vi "LarmorOptimization(SubVI).vi"(10 "Initial Larmor Frequency":dbl, 11 "Pulse Train File in":path) -> (3 "Larmor Frequency 3":dbl)   [LabVIEW 2020]
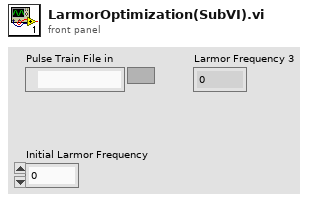
[diagram p1: front panel]
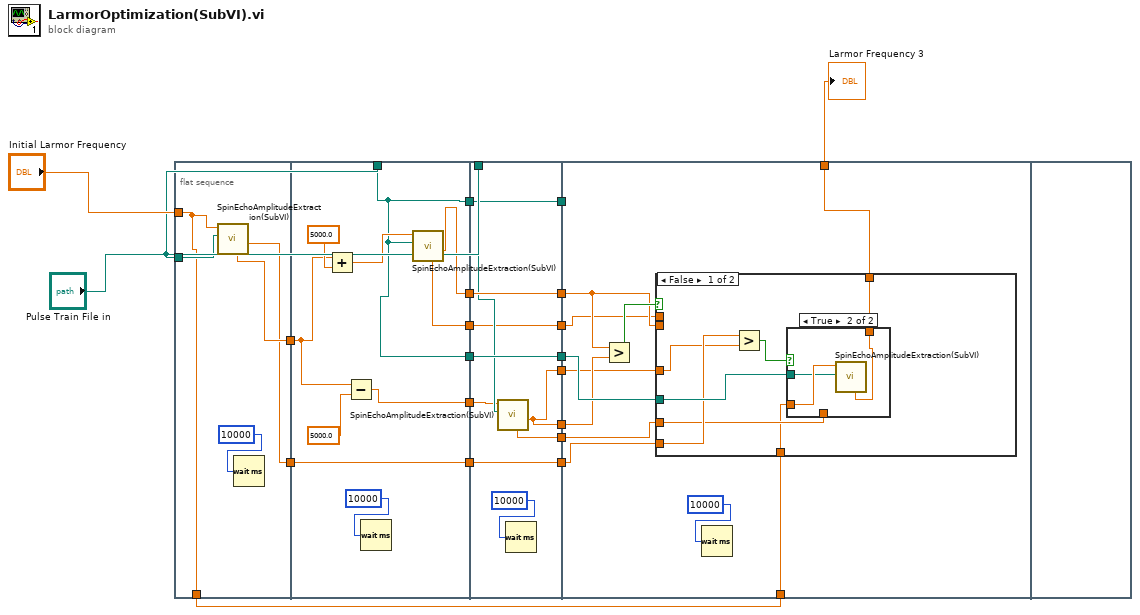
[diagram p0: block diagram]
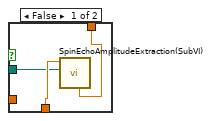
[diagram p2: hidden frame]
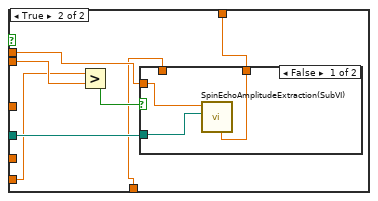
[diagram p3: hidden frame]
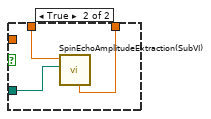
[diagram p4: hidden frame]
diagram:
  n1 = flat-sequence {
    tunnel: "Pulse Train File in" -> [w25]
    tunnel: "Initial Larmor Frequency" -> [w24]
    tunnel: [w23] -> w20
    tunnel: [w24] -> w1
    tunnel: [w21] -> w2
    tunnel: w20 -> [w34]
    tunnel: [w30] -> w19
    tunnel: "Pulse Train File in" -> [w31]
    tunnel: [w31] -> w18
    tunnel: [w31] -> w17
    tunnel: [w29] -> w16
    tunnel: [w27] -> w15
    tunnel: [w26] -> w3
    tunnel: w2 -> [w26]
    tunnel: w19 -> [w45]
    tunnel: [w45] -> w14
    tunnel: [w37] -> w13
    tunnel: w18 -> [w44]
    tunnel: [w44] -> w12
    tunnel: w17 -> [w43]
    tunnel: [w43] -> w11
    tunnel: "Pulse Train File in" -> [w42]
    tunnel: w16 -> [w41]
    tunnel: [w39] -> w10
    tunnel: w15 -> [w39]
    tunnel: [w38] -> w9
    tunnel: [w37] -> w5
    tunnel: [w36] -> w4
    tunnel: w3 -> [w36]
    tunnel: w14 -> [w47]
    tunnel: w13 -> [w54]
    tunnel: w12 -> [w55]
    tunnel: w11 -> [_]
    tunnel: w10 -> [w46]
    tunnel: w9 -> [w50]
    tunnel: [w53] -> w7
    tunnel: w5 -> [w51]
    tunnel: w4 -> [w49]
    tunnel: w1 -> [w48]
    frame #0 {
      n2 = call "SpinEchoAmplitudeExtraction(SubVI).vi"("Pulse Train File in"=w25, "Larmor Frequency in"=w24) -> ("Y value"=w21:dbl, "Larmor Frequency 3"=w23:dbl)  [unwired: 5 in, 3 out]
      n3 = Wait (ms)(milliseconds to wait=u32 10000) -> ()  [unwired: 1 out]
    }
    frame #1 {
      n4 = Add(x=w34, y=5000.0) -> (x+y=w32:dbl)
      n5 = Subtract(x=w34, y=5000.0) -> (x-y=w29:dbl)
      n6 = Wait (ms)(milliseconds to wait=u32 10000) -> ()  [unwired: 1 out]
      n7 = call "SpinEchoAmplitudeExtraction(SubVI).vi"("Pulse Train File in"=w31, "Larmor Frequency in"=w32) -> ("Y value"=w30:dbl, "Larmor Frequency 3"=w27:dbl)  [unwired: 5 in, 3 out]
    }
    frame #2 {
      n8 = call "SpinEchoAmplitudeExtraction(SubVI).vi"("Pulse Train File in"=w42, "Larmor Frequency in"=w41) -> ("Y value"=w37:dbl, "Larmor Frequency 3"=w38:dbl)  [unwired: 5 in, 3 out]
      n9 = Wait (ms)(milliseconds to wait=u32 10000) -> ()  [unwired: 1 out]
    }
    frame #3 {
      n10 = Greater?(x=w47, y=w54) -> (0:w56:bool)
      n11 = case shown="False" w56 {
        tunnel: w49 -> [w61 w73]
        tunnel: w55 -> [w62 w75]
        tunnel: w47 -> [_ w74]
        tunnel: w51 -> [w59 _]
        tunnel: [w60 w72] -> w53
        tunnel: w50 -> [w58 _]
        tunnel: w48 -> [w57 w70]
        tunnel: w46 -> [_ w71]
        frame False {
          n12 = Greater?(x=w61, y=w59) -> (0:w63:bool)
          n13 = case shown="True" w63 {
            tunnel: w62 -> [w65 w68]
            tunnel: w57 -> [_ w69]
            tunnel: [w64 w67] -> w60
            tunnel: w58 -> [w66 _]
            frame False {
              n14 = call "SpinEchoAmplitudeExtraction(SubVI).vi"("Pulse Train File in"=w65, "Larmor Frequency in"=w66) -> ("Larmor Frequency 3"=w64:dbl)  [unwired: 5 in, 4 out]
            }
            frame True {
              n15 = call "SpinEchoAmplitudeExtraction(SubVI).vi"("Pulse Train File in"=w68, "Larmor Frequency in"=w69) -> ("Larmor Frequency 3"=w67:dbl)  [unwired: 5 in, 4 out]
            }
          }
        }
        frame True {
          n16 = Greater?(x=w73, y=w74) -> (0:w76:bool)
          n17 = case shown="False" w76 {
            tunnel: w75 -> [w78 w80]
            tunnel: w71 -> [w79 _]
            tunnel: w70 -> [_ w82]
            tunnel: [w77 w81] -> w72
            frame False {
              n18 = call "SpinEchoAmplitudeExtraction(SubVI).vi"("Pulse Train File in"=w78, "Larmor Frequency in"=w79) -> ("Larmor Frequency 3"=w77:dbl)  [unwired: 5 in, 4 out]
            }
            frame True {
              n19 = call "SpinEchoAmplitudeExtraction(SubVI).vi"("Pulse Train File in"=w80, "Larmor Frequency in"=w82) -> ("Larmor Frequency 3"=w81:dbl)  [unwired: 5 in, 4 out]
            }
          }
        }
      }
      n20 = Wait (ms)(milliseconds to wait=u32 10000) -> ()  [unwired: 1 out]
    }
    frame #4 {
    }
  }
  "Larmor Frequency 3" <- w7
